vi "R Arm Initial Position.vi"(0 "Cluster":T1={"R Trans/SJC"=refnum, "R For/EJC"=refnum, "Shoulder Angle"=0.0, "Shoulder Axis"={"X"=-1.0, "Y"=0.0, "Z"=0.0}, "Elbow Angle"=0.0, "Elbow Axis"={"X"=0.0, "Y"=-1.0, "Z"=0.0}}) -> (1 "Scene.Object Out":refnum<vi>, 3 "Scene.Object Out 3":refnum<vi>)   [LabVIEW 2010]
uses:
  <vilib>/picture/3D Picture Control/NI_3D Picture Control.lvlib
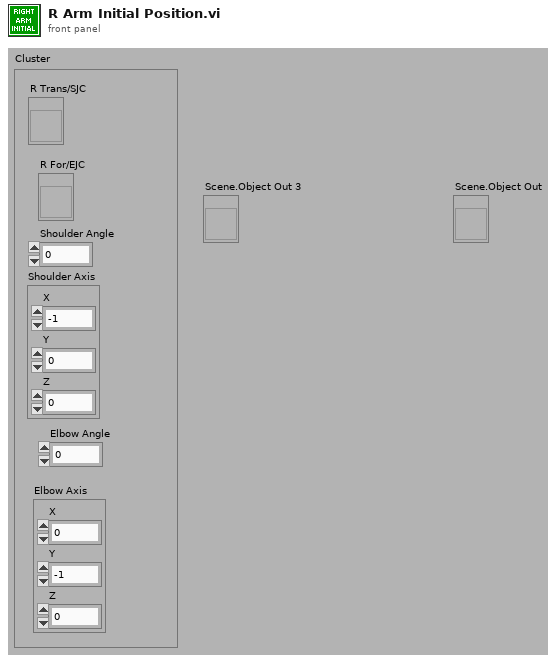
[diagram p1: front panel]
types:
  T1 = cluster{"R Trans/SJC":refnum<vi>, "R For/EJC":refnum<vi>, "Shoulder Angle":dbl, "Shoulder Axis":cluster{"X":sgl, "Y":sgl, "Z":sgl}, "Elbow Angle":dbl, "Elbow Axis":cluster{"X":sgl, "Y":sgl, "Z":sgl}}
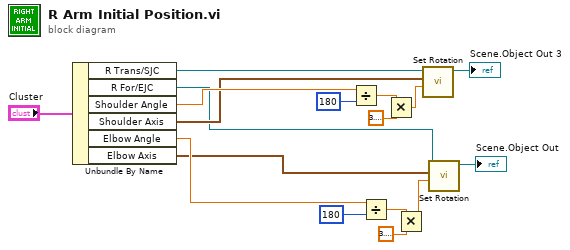
[diagram p0: block diagram]
diagram:
  n1 = Unbundle By Name("Cluster") -> ("R Trans/SJC"=w2:refnum<vi>, "R For/EJC"=w1:refnum<vi>, "Shoulder Angle"=w6:dbl, "Shoulder Axis"=w5:cluster{"X":sgl, "Y":sgl, "Z":sgl}, "Elbow Angle"=w4:dbl, "Elbow Axis"=w3:cluster{"X":sgl, "Y":sgl, "Z":sgl})
  n2 = Divide(x=w6, y=180) -> (x/y=w14:dbl)
  n3 = Divide(x=w4, y=180) -> (x/y=w9:dbl)
  n4 = Multiply(x=w14, y=3.141592653589793) -> (x*y=w12:dbl)
  n5 = Multiply(x=w9, y=3.141592653589793) -> (x*y=w11:dbl)
  n6 = call <vilib>:"Set Rotation.vi"("Angle"=w12, "Axis"=w5, "Scene Object"=w2) -> ("Rotated Scene Object"=→"Scene.Object Out 3":refnum<vi>)  [unwired: 7 in, 1 out]
  n7 = call <vilib>:"Set Rotation.vi"("Angle"=w11, "Axis"=w3, "Scene Object"=w1) -> ("Rotated Scene Object"=→"Scene.Object Out":refnum<vi>)  [unwired: 7 in, 1 out]
